vi "Initialize.vi"(6 "error in":errorcluster, 9 "RegRefAdj":i32=16 min=0 max=31 step=1) -> (0 "error out":errorcluster)   [LabVIEW 2011]
doc: "This VI performs any activity that needs to occur for proper operation of Orochi prior to powerup then powers up the unit. This activity includes initializing variables, setting variable values, running any necessary scripts, resetting the scope, etc.\n\nInputs:\n1. RegRefAdj: Value of to set RegRefAdj (0-31)."
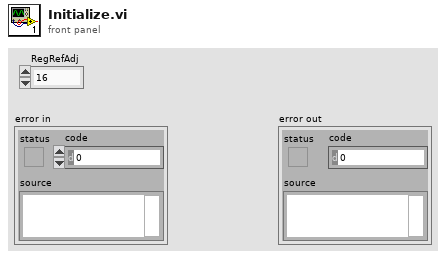
[diagram p1: front panel]
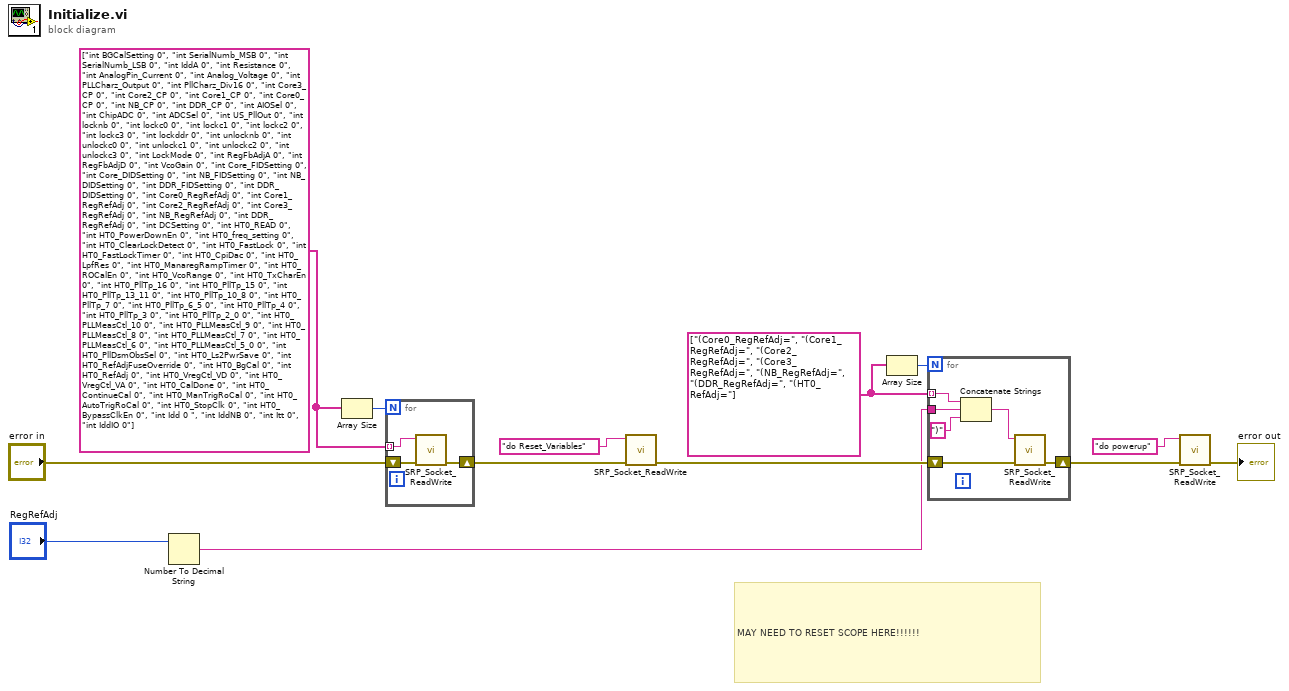
[diagram p0: block diagram]
diagram:
  w9 = string[] ["(Core0_RegRefAdj=", "(Core1_RegRefAdj=", "(Core2_RegRefAdj=", "(Core3_RegRefAdj=", "(NB_RegRefAdj=", "(DDR_RegRefAdj=", "(HT0_RefAdj="]
  w7 = string[] ["int BGCalSetting 0", "int SerialNumb_MSB 0", "int SerialNumb_LSB 0", "int IddA 0", "int Resistance 0", "int AnalogPin_Current 0", "int Analog_Voltage 0", "int PLLCharz_Output 0", "int PllCharz_Div16 0", "int Core3_CP 0", "int Core2_CP 0", "int Core1_CP 0", "int Core0_CP 0", "int NB_CP 0", "int DDR_CP 0", "int AIOSel 0", "int ChipADC 0", "int ADCSel 0", "int US_PllOut 0", "int locknb 0", "int lockc0 0", "int lockc1 0", "int lockc2 0", "int lockc3 0", "int lockddr 0", "int unlocknb 0", "int unlockc0 0", "int unlockc1 0", "int unlockc2 0", "int unlockc3 0", "int LockMode 0", "int RegFbAdjA 0", "int RegFbAdjD 0", "int VcoGain 0", "int Core_FIDSetting 0", "int Core_DIDSetting 0", "int NB_FIDSetting 0", "int NB_DIDSetting 0", "int DDR_FIDSetting 0", "int DDR_DIDSetting 0", "int Core0_RegRefAdj 0", "int Core1_RegRefAdj 0", "int Core2_RegRefAdj 0", "int Core3_RegRefAdj 0", "int NB_RegRefAdj 0", "int DDR_RegRefAdj 0", "int DCSetting 0", "int HT0_READ 0", "int HT0_PowerDownEn 0", "int HT0_freq_setting 0", "int HT0_ClearLockDetect 0", "int HT0_FastLock 0", "int HT0_FastLockTimer 0", "int HT0_CpiDac 0", "int HT0_LpfRes 0", "int HT0_ManaregRampTimer 0", "int HT0_ROCalEn 0", "int HT0_VcoRange 0", "int HT0_TxCharEn 0", "int HT0_PllTp_16 0", "int HT0_PllTp_15 0", "int HT0_PllTp_13_11 0", "int HT0_PllTp_10_8 0", "int HT0_PllTp_7 0", "int HT0_PllTp_6_5 0", "int HT0_PllTp_4 0", "int HT0_PllTp_3 0", "int HT0_PllTp_2_0 0", "int HT0_PLLMeasCtl_10 0", "int HT0_PLLMeasCtl_9 0", "int HT0_PLLMeasCtl_8 0", "int HT0_PLLMeasCtl_7 0", "int HT0_PLLMeasCtl_6 0", "int HT0_PLLMeasCtl_5_0 0", "int HT0_PllDsmObsSel 0", "int HT0_Ls2PwrSave 0", "int HT0_RefAdjFuseOverride 0", "int HT0_BgCal 0", "int HT0_RefAdj 0", "int HT0_VregCtl_VD 0", "int HT0_VregCtl_VA 0", "int HT0_CalDone 0", "int HT0_ContinueCal 0", "int HT0_ManTrigRoCal 0", "int HT0_AutoTrigRoCal 0", "int HT0_StopClk 0", "int HT0_BypassClkEn 0", "int Idd 0 ", "int IddNB 0", "int Itt 0", "int IddIO 0"]
  # "MAY NEED TO RESET SCOPE HERE!!!!!!"
  n1 = Number To Decimal String(number="RegRefAdj") -> (decimal integer string=w1:string)  [unwired: 1 in]
  n2 = Array Size(array=w7) -> (size(s)=w11:i32)
  n3 = for {
    N: w11 -> [_]
    shift-right: [w15] -> w8
    shift-left: "error in" -> [w16]
    tunnel: w7 -> [w14] mode=indexing
    n4 = call "SRP_Socket_ReadWrite.vi"("error in (no error)"=w16, "Data In"=w14) -> ("error out"=w15:errorcluster)  [unwired: 7 in, 1 out]
  }
  n5 = call "SRP_Socket_ReadWrite.vi"("error in (no error)"=w8, "Data In"="do Reset_Variables") -> ("error out"=w6:errorcluster)  [unwired: 7 in, 1 out]
  n6 = Array Size(array=w9) -> (size(s)=w10:i32)
  n7 = for {
    N: w10 -> [_]
    tunnel: w9 -> [w22] mode=indexing
    tunnel: w1 -> [w21]
    shift-right: [w20] -> w5
    shift-left: w6 -> [w19]
    n8 = Concatenate Strings(w22, w21, ")") -> (w17:string)
    n9 = call "SRP_Socket_ReadWrite.vi"("error in (no error)"=w19, "Data In"=w17) -> ("error out"=w20:errorcluster)  [unwired: 7 in, 1 out]
  }
  n10 = call "SRP_Socket_ReadWrite.vi"("error in (no error)"=w5, "Data In"="do powerup") -> ("error out"=→"error out":errorcluster)  [unwired: 7 in, 1 out]
